vi "Write Msg Input.vi"(10 "Msg Input":refnum<class "Msg Input.lvclass">, 11 "TEMPLATE Msg in":refnum<class "TEMPLATE Msg.lvclass">) -> (3 "TEMPLATE Msg out":refnum<class "TEMPLATE Msg.lvclass">)   [LabVIEW 2025, in "_Template.lvlib" / "Templates.lvlib" / "TEMPLATE Msg.lvlib" / "TEMPLATE Msg.lvlib" / "TEMPLATE Msg.lvclass"]
uses:
  TEMPLATE Msg.lvclass
  TEMPLATE Msg.lvclass/TEMPLATE Msg.ctl
  jettl/jettl/Msg Input/Msg Input.lvclass
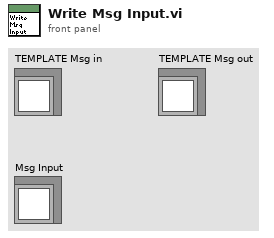
[diagram p1: front panel]
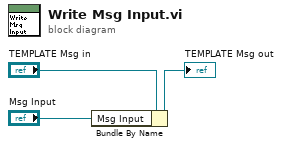
[diagram p0: block diagram]
diagram:
  n1 = Bundle By Name(cluster="TEMPLATE Msg in", "Msg Input"="Msg Input") -> (→"TEMPLATE Msg out":refnum<class "TEMPLATE Msg.lvclass">)
